vi "manual test UI.vi"(8 "error in (no error)":errorcluster caption="Fehler (Eingang, kein Fehler)", 11 "Burst Eingang":refnum<class "Burst.lvclass"> caption="DNL_LabVIEW Object in") -> (0 "error out":errorcluster caption="Fehler (Ausgang)", 1 "abbrechen":bool, 2 "Parameters":u32[](array[numeric]), 3 "Burst Ausgang":refnum<class "Burst.lvclass"> caption="DNL_LabVIEW Object out")   [LabVIEW 2013, in "Burst.lvclass"]
uses:
  Burst.lvclass
  Polaritaet.ctl
  lib/Utilities.lvlib
panel:
  in  "#OfAmps":u32=1 min=1 max=4 step=1
  in  "Amplituden (200 - 4200V) 4":u32=200 min=200 max=4200 step=10
  in  "Amplituden (200 - 4200V) 3":u32=200 min=200 max=4200 step=10
  in  "Amplituden (200 - 4200V) 2":u32=200 min=200 max=4200 step=10
  in  "Testbeschreibung":string
  in  "Testdauer (1s - 10000s)":u32=1 min=1 max=1000
  in  "Burstperiode (10ms - 2400ms)":u32=10 min=10 max=2400
  in  "Burstdauer (1 - 130ms)":u32=1 min=1 max=130
  in  "Spike-Frequenz (500Hz - 100000Hz)":u32=500 min=500 max=100000
  in  "Amplituden (200 - 4200V)":u32=200 min=200 max=4200 step=10
  in  "Einkopplung":bool
  in  "Polarität":T1
  in  "ok":bool
  in  "abbrechen 2":bool
  # "bis zu 4 verschiedne Amplituden können angegebn werden"
  # "Polarität"
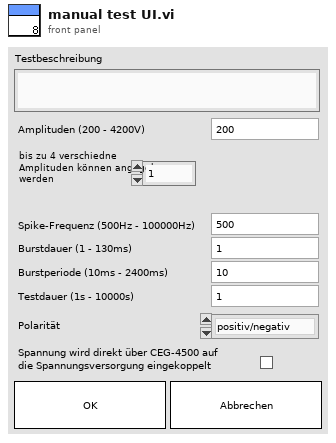
[diagram p1: front panel]
types:
  T1 = typedef "Burst.lvclass/Polaritaet.ctl" = enum16{"positiv/negativ", "negativ", "positiv"}
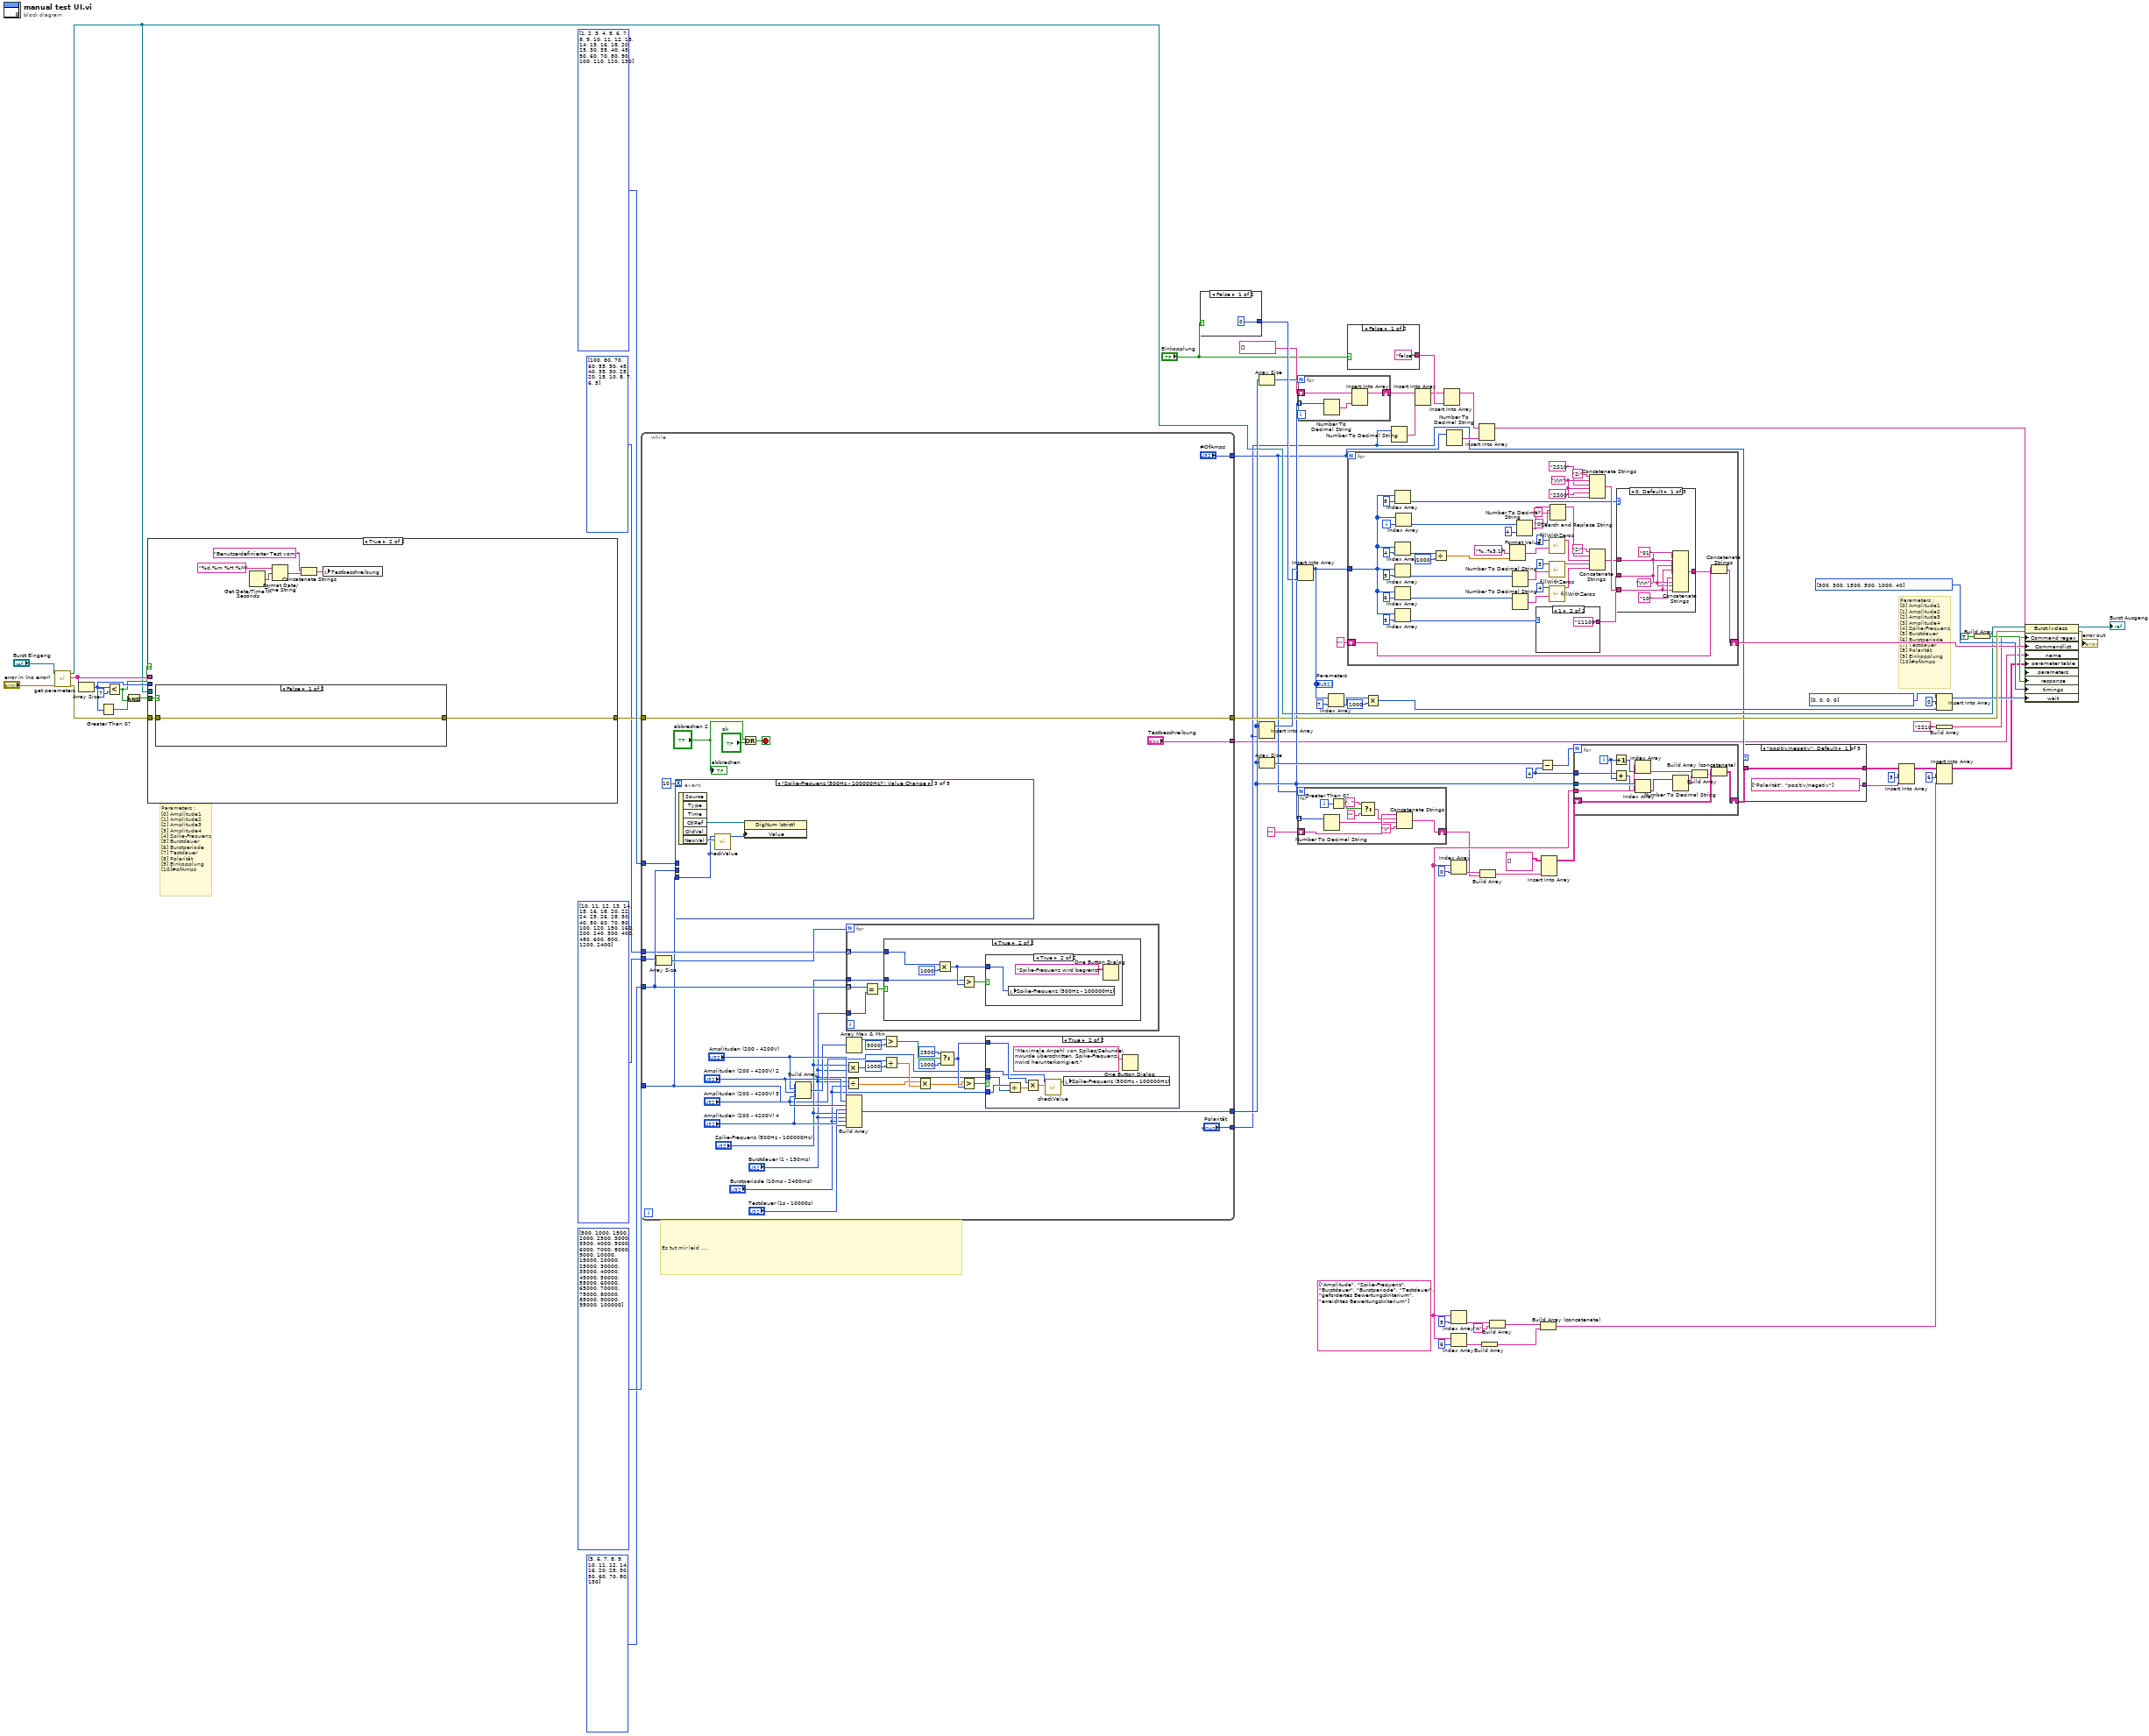
[diagram p0: block diagram]
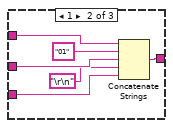
[diagram p2: hidden frame]
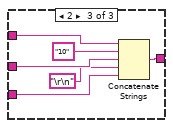
[diagram p3: hidden frame]
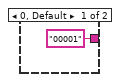
[diagram p4: hidden frame]
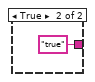
[diagram p5: hidden frame]
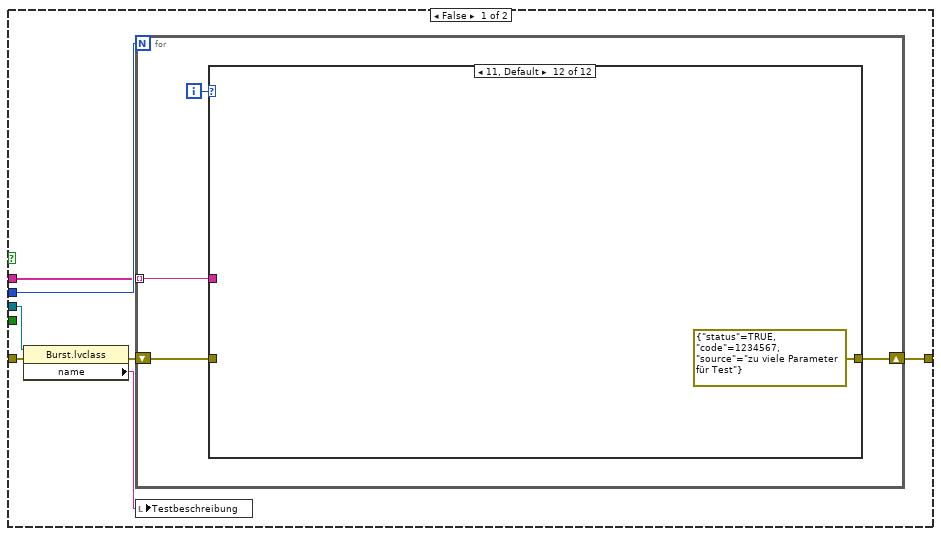
[diagram p6: hidden frame]
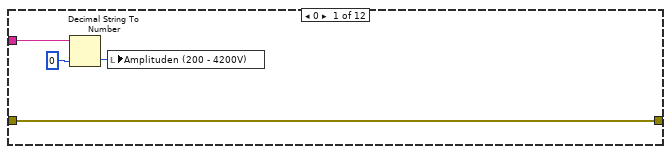
[diagram p7: hidden frame]
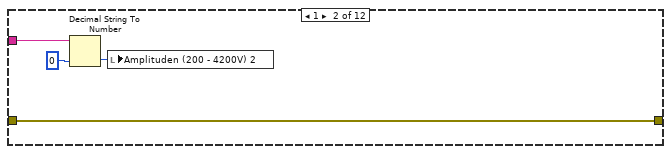
[diagram p8: hidden frame]
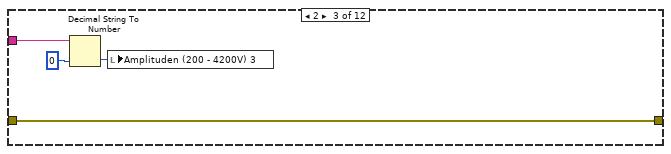
[diagram p9: hidden frame]
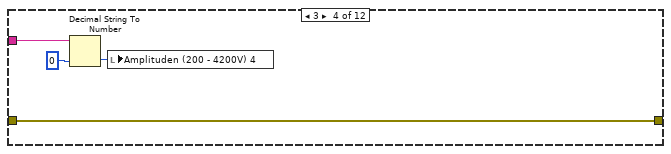
[diagram p10: hidden frame]
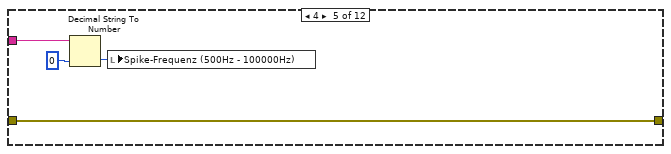
[diagram p11: hidden frame]
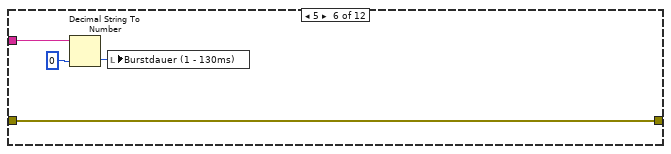
[diagram p12: hidden frame]
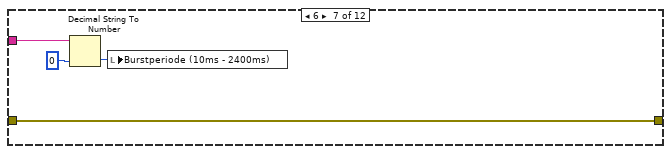
[diagram p13: hidden frame]
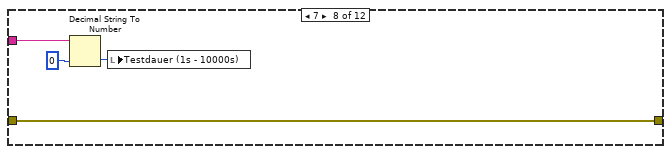
[diagram p14: hidden frame]
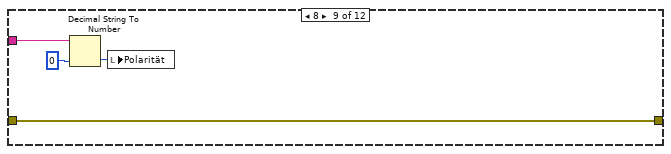
[diagram p15: hidden frame]
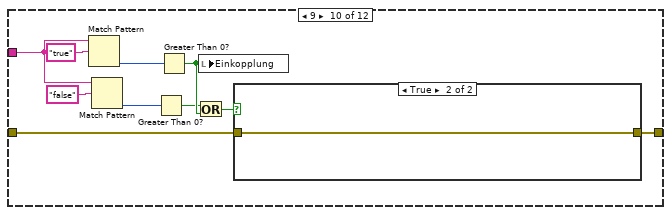
[diagram p16: hidden frame]
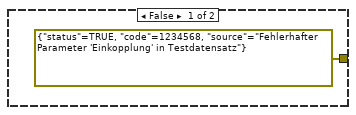
[diagram p17: hidden frame]
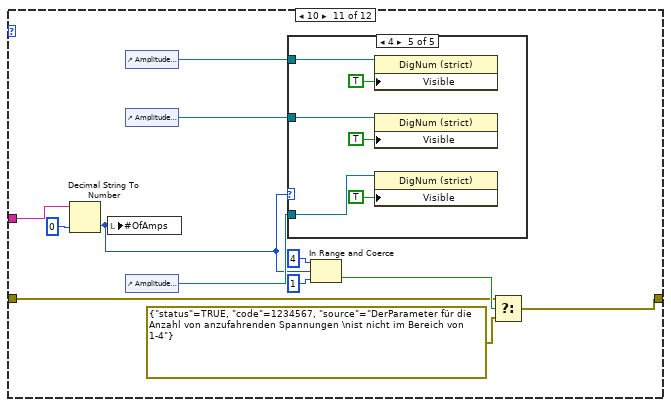
[diagram p18: hidden frame]
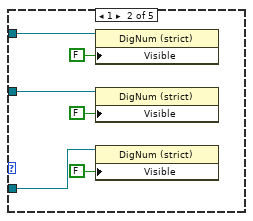
[diagram p20: hidden frame]
diagram:
  w24 = 4 ("y")
  w22 = string[] ["Amplitude", "Spike-Frequenz", "Burstdauer", "Burstperiode", "Testdauer", "gefordertes Bewertungskriterium", "erreichtes Bewertungskriterium"]
  # "Parameters :\n[0] Amplitude1\n[1] Amplitude2\n[2] Amplitude3\n[3] Amplitude4\n[4] Spike-Frequenz\n[5] Burstdauer\n[6] Burstperiode\n[7] Testdauer\n[8] Polarität\n[9] Einkopplung\n[10]#ofAmps"
  # "Parameters :\n[0] Amplitude1\n[1] Amplitude2\n[2] Amplitude3\n[3] Amplitude4\n[4] Spike-Frequenz\n[5] Burstdauer\n[6] Burstperiode\n[7] Testdauer\n[8] Polarität\n[9] Einkopplung\n[10]#ofAmps"
  # "Es tut mir leid ...."
  n1 = call-dynamic "get parameters.vi"("error in (no error)"="error in (no error)", "TestInterface (Eingang)"="Burst Eingang") -> ("error out"=w57:errorcluster, "parameters"=w58:string[], "TestInterface (Ausgang)"=w29:refnum<class "Burst.lvclass">)  [unwired: 7 in]
  n2 = Array Size(array=w58) -> (size(s)=w40:i32)
  n3 = Greater Than 0?(x=w40) -> (x > 0?=w39:bool)
  n4 = Less?(x=w40, y=7) -> (x < y?=w38:bool)
  n5 = And(x=w39, y=w38) -> (x .and. y?=w37:bool)
  n6 = case shown="True" w38 {
    tunnel: w40 -> [w83 _]
    tunnel: w58 -> [w82 _]
    tunnel: w57 -> [w79 w175]
    tunnel: [w81 w173] -> w56
    tunnel: w37 -> [_ w174]
    tunnel: w29 -> [w80 _]
    frame False {
      n7 = property class="Burst.lvclass"(reference=w80, error in=w79) -> (error out=w78:errorcluster, "name"=w77:string)  [unwired: 1 out]
      n8 = for {
        N: w83 -> [_]
        tunnel: w82 -> [w86] mode=indexing
        shift-right: [w85] -> w81
        shift-left: w78 -> [w84]
        i -> [w87]
        n9 = case shown="11, Default" w87 {
          tunnel: w86 -> [w91 w95 w99 w103 w105 w109 w113 w117 w121 w124 w146 _]
          tunnel: w84 -> [w88 w92 w96 w100 w104 w108 w112 w116 w120 w126 w142 _]
          tunnel: [w88 w92 w96 w100 w104 w108 w112 w116 w120 w128 w141 errorcluster {"status"=TRUE, "code"=1234567, "source"="zu viele Parameter für Test"} ("error constant")] -> w85
          frame 0 {
            n10 = Decimal String To Number(string=w91, default (0L)=u32 0 ("default (0 I32)")) -> (number=w90:u32)  [unwired: 1 in, 1 out]
            n11 = local write "Amplituden (200 - 4200V)"(w90) -> ()
          }
          frame 1 {
            n12 = Decimal String To Number(string=w95, default (0L)=u32 0 ("default (0 I32)")) -> (number=w94:u32)  [unwired: 1 in, 1 out]
            n13 = local write "Amplituden (200 - 4200V) 2"(w94) -> ()
          }
          frame 2 {
            n14 = Decimal String To Number(string=w99, default (0L)=u32 0 ("default (0 I32)")) -> (number=w98:u32)  [unwired: 1 in, 1 out]
            n15 = local write "Amplituden (200 - 4200V) 3"(w98) -> ()
          }
          frame 3 {
            n16 = Decimal String To Number(string=w103, default (0L)=u32 0 ("default (0 I32)")) -> (number=w102:u32)  [unwired: 1 in, 1 out]
            n17 = local write "Amplituden (200 - 4200V) 4"(w102) -> ()
          }
          frame 4 {
            n18 = Decimal String To Number(string=w105, default (0L)=u32 0 ("default (0 I32)")) -> (number=w106:u32)  [unwired: 1 in, 1 out]
            n19 = local write "Spike-Frequenz (500Hz - 100000Hz)"(w106) -> ()
          }
          frame 5 {
            n20 = Decimal String To Number(string=w109, default (0L)=u32 0 ("default (0 I32)")) -> (number=w110:u32)  [unwired: 1 in, 1 out]
            n21 = local write "Burstdauer (1 - 130ms)"(w110) -> ()
          }
          frame 6 {
            n22 = Decimal String To Number(string=w113, default (0L)=u32 0 ("default (0 I32)")) -> (number=w114:u32)  [unwired: 1 in, 1 out]
            n23 = local write "Burstperiode (10ms - 2400ms)"(w114) -> ()
          }
          frame 7 {
            n24 = Decimal String To Number(string=w117, default (0L)=u32 0 ("default (0 I32)")) -> (number=w118:u32)  [unwired: 1 in, 1 out]
            n25 = local write "Testdauer (1s - 10000s)"(w118) -> ()
          }
          frame 8 {
            n26 = Decimal String To Number(string=w121, default (0L)=u32 0 ("default (0 I32)")) -> (number=w122:u32)  [unwired: 1 in, 1 out]
            n27 = local write "Polarität"(w122) -> ()
          }
          frame 9 {
            n28 = Match Pattern(string=w124, regular expression="true") -> (offset past match=w132:i32)  [unwired: 1 in, 3 out]
            n29 = Match Pattern(string=w124, regular expression="false") -> (offset past match=w130:i32)  [unwired: 1 in, 3 out]
            n30 = Greater Than 0?(x=w130) -> (x > 0?=w127:bool)
            n31 = Greater Than 0?(x=w132) -> (x > 0?=w129:bool)
            n32 = Or(x=w127, y=w129) -> (x .or. y?=w125:bool)
            n33 = local write "Einkopplung"(w129) -> ()
            n34 = case shown="True" w125 {
              tunnel: [errorcluster {"status"=TRUE, "code"=1234568, "source"="Fehlerhafter Parameter 'Einkopplung' in Testdatensatz"} ("error constant") w135] -> w128
              tunnel: w126 -> [_ w135]
              frame False {
              }
              frame True {
              }
            }
          }
          frame 10 {
            n35 = Decimal String To Number(string=w146, default (0L)=u32 0 ("default (0 I32)")) -> (number=w136:u32)  [unwired: 1 in, 1 out]
            n36 = local write "#OfAmps"(w136) -> ()
            n37 = control-ref of="Amplituden (200 - 4200V) 4"() -> (w137:refnum<vi>)
            n38 = control-ref of="Amplituden (200 - 4200V) 2"() -> (w139:refnum<vi>)
            n39 = control-ref of="Amplituden (200 - 4200V) 3"() -> (w138:refnum<vi>)
            n40 = case shown="4" w136 {
              tunnel: w139 -> [_ w153 w159 w165 w171]
              tunnel: w138 -> [_ w149 w155 w161 w167]
              tunnel: w137 -> [_ w148 w154 w160 w166]
              frame 0, Default {
              }
              frame 1 {
                n41 = property class="DigNum (strict)"(reference=w148, "Visible"=FALSE) -> ()  [unwired: 1 in, 2 out]
                n42 = property class="DigNum (strict)"(reference=w153, "Visible"=FALSE) -> ()  [unwired: 1 in, 2 out]
                n43 = property class="DigNum (strict)"(reference=w149, "Visible"=FALSE) -> ()  [unwired: 1 in, 2 out]
              }
              frame 2 {
                n44 = property class="DigNum (strict)"(reference=w154, "Visible"=FALSE) -> ()  [unwired: 1 in, 2 out]
                n45 = property class="DigNum (strict)"(reference=w159, "Visible"=TRUE) -> ()  [unwired: 1 in, 2 out]
                n46 = property class="DigNum (strict)"(reference=w155, "Visible"=FALSE) -> ()  [unwired: 1 in, 2 out]
              }
              frame 3 {
                n47 = property class="DigNum (strict)"(reference=w160, "Visible"=FALSE) -> ()  [unwired: 1 in, 2 out]
                n48 = property class="DigNum (strict)"(reference=w165, "Visible"=TRUE) -> ()  [unwired: 1 in, 2 out]
                n49 = property class="DigNum (strict)"(reference=w161, "Visible"=TRUE) -> ()  [unwired: 1 in, 2 out]
              }
              frame 4 {
                n50 = property class="DigNum (strict)"(reference=w166, "Visible"=TRUE) -> ()  [unwired: 1 in, 2 out]
                n51 = property class="DigNum (strict)"(reference=w171, "Visible"=TRUE) -> ()  [unwired: 1 in, 2 out]
                n52 = property class="DigNum (strict)"(reference=w167, "Visible"=TRUE) -> ()  [unwired: 1 in, 2 out]
              }
            }
            n53 = In Range and Coerce(upper limit=u32 4, x=w136, lower limit=u32 1) -> (In Range?=w143:bool)  [unwired: 1 out]
            n54 = Select(t=w142, s=w143, f=errorcluster {"status"=TRUE, "code"=1234567, "source"="DerParameter für die Anzahl von anzufahrenden Spannungen \nist nicht im Bereich von 1-4"} ("error constant")) -> (s? t:f=w141:errorcluster)
          }
          frame 11, Default {
          }
        }
      }
      n55 = local write "Testbeschreibung"(w77) -> ()
    }
    frame True {
      n56 = case shown="False" w174 {
        tunnel: w175 -> [w181 _]
        tunnel: [w181 errorcluster {"status"=TRUE, "code"=123458, "source"="Der Parametersatz für den aktuellen Test ist unvollständig und\nkonnte nicht geladen werden"} ("error constant")] -> w173
        frame False {
        }
        frame True {
        }
      }
      n57 = Get Date/Time In Seconds() -> (seconds since 1Jan1904=w180:timestamp)
      n58 = Format Date/Time String(time format string (%c)="%d.%m %H:%M" ("Zeitformatierungs-String (%c)"), seconds (now)=w180) -> (date/time string=w177:string)  [unwired: 1 in]
      n59 = Concatenate Strings("Benutzerdefinierter Test vom " ("name"), w177) -> (w176:string)
      n60 = local write "Testbeschreibung"(w176) -> ()
    }
  }
  n61 = while {
    tunnel: [w214] -> w23
    tunnel: u32[] [10, 11, 12, 13, 14, 15, 16, 18, 20, 22, 24, 25, 26, 28, 30, 40, 50, 60, 70, 80, 100, 120, 150, 160, 200, 240, 300, 400, 480, 600, 800, 1200, 2400] -> [w213]
    tunnel: u32[] [500, 1000, 1500, 2000, 2500, 3000, 3500, 4000, 5000, 6000, 7000, 8000, 9000, 10000, 15000, 20000, 25000, 30000, 35000, 40000, 45000, 50000, 55000, 60000, 65000, 70000, 75000, 80000, 85000, 90000, 95000, 100000] -> [w185]
    tunnel: u32[] [1, 2, 3, 4, 5, 6, 7, 8, 9, 10, 11, 12, 13, 14, 15, 16, 18, 20, 25, 30, 35, 40, 45, 50, 60, 70, 80, 90, 100, 110, 120, 130] -> [w212]
    tunnel: w56 -> [w210]
    tunnel: [w210] -> w49
    tunnel: ["#OfAmps"] -> w5
    tunnel: ["Polarität"] -> w4
    tunnel: ["Testbeschreibung"] -> w3
    tunnel: u32[] [100, 80, 70, 60, 55, 50, 45, 40, 35, 30, 25, 20, 15, 10, 8, 7, 6, 5] -> [w204]
    tunnel: u32[] [5, 6, 7, 8, 9, 10, 11, 12, 14, 16, 20, 25, 30, 50, 60, 70, 80, 130] -> [w205]
    stop <- w218 stop-if-true
    n62 = Array Size(array=w205) -> (size(s)=w206:i32)
    n63 = event shown="[2] \"Spike-Frequenz (500Hz - 100000Hz)\": Value Change" {
      selector: _ -> [_ _ _ _ _]
      dyn-events: _ -> [_ _ _ _ _]
      timeout: 10 -> [_ _ _ _ _]
      tunnel: w213 -> [w242 _ _ _ _]
      tunnel: w185 -> [_ _ w243 _ _]
      tunnel: w212 -> [_ _ _ _ w275]
      event "Burstperiode (10ms - 2400ms)": Value Change {
        n64 = event-data() -> ("CtlRef"=w240:refnum<vi>, "NewVal"=w241:u32)  [unwired: 1 in, 4 out]
        n65 = call "checkValue.vi"("Value"=w241, "Array of valid Values"=w242) -> ("new Value"=w239:u32)  [unwired: 7 in]
        n66 = property class="DigNum (strict)"(reference=w240, "Value"=w239) -> ()  [unwired: 1 in, 2 out]
      }
      event Timeout {
        n67 = event-data() -> ()  [unwired: 1 in, 3 out]
      }
      event "Spike-Frequenz (500Hz - 100000Hz)": Value Change {
        n68 = event-data() -> ("CtlRef"=w245:refnum<vi>, "NewVal"=w244:u32)  [unwired: 1 in, 4 out]
        n69 = call "checkValue.vi"("Value"=w244, "Array of valid Values"=w243) -> ("new Value"=w246:u32)  [unwired: 7 in]
        n70 = property class="DigNum (strict)"(reference=w245, "Value"=w246) -> ()  [unwired: 1 in, 2 out]
      }
      event "#OfAmps": Value Change {
        n71 = event-data() -> ("NewVal"=w250:u32)  [unwired: 1 in, 5 out]
        n72 = control-ref of="Amplituden (200 - 4200V) 4"() -> (w247:refnum<vi>)
        n73 = control-ref of="Amplituden (200 - 4200V) 3"() -> (w248:refnum<vi>)
        n74 = control-ref of="Amplituden (200 - 4200V) 2"() -> (w249:refnum<vi>)
        n75 = case shown="4" w250 {
          tunnel: w249 -> [_ w256 w262 w268 w274]
          tunnel: w248 -> [_ w252 w258 w264 w270]
          tunnel: w247 -> [_ w251 w257 w263 w269]
          frame 0, Default {
          }
          frame 1 {
            n76 = property class="DigNum (strict)"(reference=w251, "Visible"=FALSE) -> ()  [unwired: 1 in, 2 out]
            n77 = property class="DigNum (strict)"(reference=w252, "Visible"=FALSE) -> ()  [unwired: 1 in, 2 out]
            n78 = property class="DigNum (strict)"(reference=w256, "Visible"=FALSE) -> ()  [unwired: 1 in, 2 out]
          }
          frame 2 {
            n79 = property class="DigNum (strict)"(reference=w257, "Visible"=FALSE) -> ()  [unwired: 1 in, 2 out]
            n80 = property class="DigNum (strict)"(reference=w258, "Visible"=FALSE) -> ()  [unwired: 1 in, 2 out]
            n81 = property class="DigNum (strict)"(reference=w262, "Visible"=TRUE) -> ()  [unwired: 1 in, 2 out]
          }
          frame 3 {
            n82 = property class="DigNum (strict)"(reference=w263, "Visible"=FALSE) -> ()  [unwired: 1 in, 2 out]
            n83 = property class="DigNum (strict)"(reference=w264, "Visible"=TRUE) -> ()  [unwired: 1 in, 2 out]
            n84 = property class="DigNum (strict)"(reference=w268, "Visible"=TRUE) -> ()  [unwired: 1 in, 2 out]
          }
          frame 4 {
            n85 = property class="DigNum (strict)"(reference=w269, "Visible"=TRUE) -> ()  [unwired: 1 in, 2 out]
            n86 = property class="DigNum (strict)"(reference=w270, "Visible"=TRUE) -> ()  [unwired: 1 in, 2 out]
            n87 = property class="DigNum (strict)"(reference=w274, "Visible"=TRUE) -> ()  [unwired: 1 in, 2 out]
          }
        }
      }
      event "Burstdauer (1 - 130ms)": Value Change {
        n88 = event-data() -> ("CtlRef"=w277:refnum<vi>, "NewVal"=w276:u32)  [unwired: 1 in, 4 out]
        n89 = call "checkValue.vi"("Value"=w276, "Array of valid Values"=w275) -> ("new Value"=w278:u32)  [unwired: 7 in]
        n90 = property class="DigNum (strict)"(reference=w277, "Value"=w278) -> ()  [unwired: 1 in, 2 out]
      }
    }
    n91 = Or(x="abbrechen 2", y="ok") -> (x .or. y?=w218:bool)
    n92 = Build Array("Amplituden (200 - 4200V) 4", "Amplituden (200 - 4200V)", "Amplituden (200 - 4200V) 2", "Amplituden (200 - 4200V) 3") -> (w199:u32[])
    n93 = Multiply(x="Spike-Frequenz (500Hz - 100000Hz)", y="Burstdauer (1 - 130ms)") -> (x*y=w190:u32)
    n94 = Divide(x="Burstdauer (1 - 130ms)", y="Burstperiode (10ms - 2400ms)") -> (x/y=w193:dbl)
    n95 = for {
      N: w206 -> [_]
      tunnel: w205 -> [w231] mode=indexing
      tunnel: "Burstdauer (1 - 130ms)" -> [w230]
      tunnel: w204 -> [w228] mode=indexing
      tunnel: "Spike-Frequenz (500Hz - 100000Hz)" -> [w227]
      n96 = Equal?(x=w231, y=w230) -> (x = y?=w229:bool)
      n97 = case shown="True" w229 {
        tunnel: w228 -> [_ w236]
        tunnel: w227 -> [_ w232]
        frame False {
        }
        frame True {
          n98 = Multiply(x=w236, y=u32 1000) -> (x*y=w233:u32)
          n99 = Greater?(x=w232, y=w233) -> (0:w234:bool)
          n100 = case shown="True" w234 {
            tunnel: w233 -> [_ w238]
            frame False {
            }
            frame True {
              n101 = local write "Spike-Frequenz (500Hz - 100000Hz)"(w238) -> ()
              n102 = One Button Dialog(message="Spike-Frequenz wird begrenzt") -> ()  [unwired: 1 in, 1 out]
            }
          }
        }
      }
    }
    n103 = Array Max & Min(array=w199) -> (max value=w198:u32)  [unwired: 3 out]
    n104 = Build Array("Amplituden (200 - 4200V)", "Amplituden (200 - 4200V) 2", "Amplituden (200 - 4200V) 3", "Amplituden (200 - 4200V) 4", "Spike-Frequenz (500Hz - 100000Hz)", "Burstdauer (1 - 130ms)", "Burstperiode (10ms - 2400ms)", "Testdauer (1s - 10000s)") -> (w214:u32[])
    n105 = Greater?(x=w198, y=u32 3000) -> (0:w196:bool)
    n106 = Divide(x=w190, y=u32 1000) -> (x/y=w191:dbl)
    n107 = Multiply(x=w193, y=w191) -> (x*y=w188:dbl)
    n108 = Select(t=u32 2500, s=w196, f=u32 1000) -> (s? t:f=w186:u32)
    n109 = Greater?(x=w188, y=w186) -> (0:w187:bool)
    n110 = case shown="True" w187 {
      tunnel: w186 -> [_ w225]
      tunnel: "Burstdauer (1 - 130ms)" -> [_ w219]
      tunnel: "Burstperiode (10ms - 2400ms)" -> [_ w220]
      tunnel: w185 -> [_ w223]
      frame False {
      }
      frame True {
        n111 = Divide(x=w220, y=w219) -> (x/y=w224:dbl)
        n112 = Multiply(x=w225, y=w224) -> (x*y=w221:dbl)
        n113 = call "checkValue.vi"("Value"=w221, "Array of valid Values"=w223) -> ("new Value"=w222:u32)  [unwired: 7 in]
        n114 = local write "Spike-Frequenz (500Hz - 100000Hz)"(w222) -> ()
        n115 = One Button Dialog(message="Maximale Anzahl von Spikes/Sekunde\nwurde überschritten. Spike-Frequenz\nwird herunterkorrigiert.") -> ()  [unwired: 1 in, 1 out]
      }
    }
    "abbrechen" <- "abbrechen 2"
  }
  n116 = case shown="False" "Einkopplung" {
    tunnel: [u32 0 u32 1] -> w75
    frame False {
    }
    frame True {
    }
  }
  n117 = Array Size(array=w23) -> (size(s)=w33:i32)
  n118 = Insert Into Array(array=w23, new element=w4) -> (w76:u32[])  [unwired: 1 in]
  n119 = Array Size(array=w23) -> (size(s)=w26:i32)
  n120 = for {
    N: w33 -> [_]
    tunnel: w23 -> [w284] mode=indexing
    shift-right: [w281] -> w10
    shift-left: string[] [] -> [w282]
    n121 = Number To Decimal String(number=w284) -> (decimal integer string=w283:string)  [unwired: 1 in]
    n122 = Insert Into Array(array=w282, new element=w283) -> (w281:string[])  [unwired: 1 in]
  }
  n123 = Insert Into Array(array=w76, new element=w75) -> (w27:u32[])  [unwired: 1 in]
  "Parameters" <- w27
  n124 = for {
    N: w5 -> [_]
    tunnel: w23 -> [w294] mode=indexing
    shift-right: [w285] -> w19
    shift-left: "" -> [w289]
    i -> [w293]
    n125 = Number To Decimal String(number=w294) -> (decimal integer string=w287:string)  [unwired: 1 in]
    n126 = Greater Than 0?(x=w293) -> (x > 0?=w292:bool)
    n127 = Select(t=", ", s=w292, f="") -> (s? t:f=w288:string)
    n128 = Concatenate Strings(w289, w288, w287, "V" ("string")) -> (w285:string)
  }
  n129 = Index Array(array=w27, index=7) -> (element=w53:u32)
  n130 = case shown="False" "Einkopplung" {
    tunnel: ["false" "true"] -> w30
    frame False {
    }
    frame True {
    }
  }
  n131 = for {
    N: w5 -> [_]
    tunnel: w27 -> [w301]
    shift-right: [w300] -> w46
    shift-left: "" -> [w299]
    i -> [w297]
    w336 = "\r\n"
    n132 = Index Array(array=w301, index=8) -> (element=w330:u32)
    n133 = Index Array(array=w301, index=4) -> (element=w310:u32)
    n134 = Index Array(array=w301, index=5) -> (element=w318:u32)
    n135 = Index Array(array=w301, index=6) -> (element=w324:u32)
    n136 = Index Array(array=w301, index=9) -> (element=w329:u32)
    n137 = Index Array(array=w301, index=w297) -> (element=w303:u32)
    n138 = Divide(x=w310, y=u32 1000) -> (x/y=w312:dbl)
    n139 = Format Value(format string="%.;%3.1f", value (0)=w312) -> (output string=w315:string)  [unwired: 1 in]
    n140 = Number To Decimal String(number=w318) -> (decimal integer string=w319:string)  [unwired: 1 in]
    n141 = Number To Decimal String(number=w324) -> (decimal integer string=w323:string)  [unwired: 1 in]
    n142 = Number To Decimal String(number=w303, width (-)=i16 4) -> (decimal integer string=w305:string)
    n143 = case shown="1" w329 {
      tunnel: ["00001" "11100"] -> w332
      frame 0, Default {
      }
      frame 1 {
      }
    }
    n144 = call "fillWithZeros.vi"("string in"=w315, "width"=5 ("x")) -> ("string out"=w316:string)  [unwired: 9 in]
    n145 = call "fillWithZeros.vi"("string in"=w319, "width"=3) -> ("string out"=w321:string)  [unwired: 9 in]
    n146 = call "fillWithZeros.vi"("string in"=w323, "width"=4) -> ("string out"=w326:string)  [unwired: 9 in]
    n147 = Search and Replace String(input string=w305, search string=" ", replace string="0" ("replace string (\"\")")) -> (result string=w308:string)  [unwired: 5 in, 3 out]
    n148 = Concatenate Strings("2i" ("String"), w336, "2S10", w336, "2S00", w336) -> (w337:string)
    n149 = Concatenate Strings("2I", w308, w316, w321, w326) -> (w331:string)
    n150 = case shown="0, Default" w330 {
      tunnel: w331 -> [w342 w350 w356]
      tunnel: w332 -> [w340 w348 w355]
      tunnel: [w343 w347 w353] -> w298
      tunnel: w337 -> [w339 w345 w351]
      frame 0, Default {
        w338 = "\r\n"
        n151 = Concatenate Strings(w342, "01" ("string"), w340, w338, w339, w342, "10" ("string"), w340, w338, w339) -> (w343:string)
      }
      frame 1 {
        n152 = Concatenate Strings(w350, "01" ("string"), w348, "\r\n", w345) -> (w347:string)
      }
      frame 2 {
        n153 = Concatenate Strings(w356, "10" ("string"), w355, "\r\n", w351) -> (w353:string)
      }
    }
    n154 = Concatenate Strings(w299, w298) -> (w300:string)
  }
  n155 = Multiply(x=w53, y=u32 1000) -> (x*y=w55:u32)
  n156 = Number To Decimal String(number=w4) -> (decimal integer string=w9:string)  [unwired: 1 in]
  n157 = Insert Into Array(array=w10, new element=w9) -> (w11:string[])  [unwired: 1 in]
  n158 = Insert Into Array(array=w11, new element=w30) -> (w7:string[])  [unwired: 1 in]
  n159 = Number To Decimal String(number=w5) -> (decimal integer string=w8:string)  [unwired: 1 in]
  n160 = Index Array(array=w22, index=0) -> (element=w20:string)
  n161 = Index Array(array=w22, index=5 ("Index")) -> (element=w65:string)
  n162 = Index Array(array=w22, index=6 ("Index")) -> (element=w66:string)
  n163 = Insert Into Array(array=w7, new element=w8) -> (w6:string[])  [unwired: 1 in]
  n164 = Build Array(w20, w19) -> (w14:string[])
  n165 = Build Array(w66) -> (w16:string[])
  n166 = Build Array(w65, "A" ("Element")) -> (w17:string[])
  n167 = Subtract(x=w26, y=w24) -> (x-y=w25:i32)
  n168 = Build Array (concatenate)(w17, w16) -> (w15:string[])
  n169 = Insert Into Array(array=string[][] [], new element=w14) -> (w12:string[][])  [unwired: 2 in]
  n170 = for {
    N: w25 -> [_]
    shift-right: [w367] -> w71
    shift-left: w12 -> [w369]
    tunnel: w23 -> [w366]
    tunnel: w24 -> [w364]
    tunnel: w22 -> [w363]
    i -> [w359]
    n171 = Increment(x=w359) -> (x+1=w360:i32)
    n172 = Add(x=w364, y=w359) -> (x+y=w362:i32)
    n173 = Index Array(array=w363, index=w360) -> (element=w361:string)
    n174 = Index Array(array=w366, index=w362) -> (element=w365:u32)
    n175 = Number To Decimal String(number=w365) -> (decimal integer string=w370:string)  [unwired: 1 in]
    n176 = Build Array(w361, w370) -> (w368:string[])
    n177 = Build Array (concatenate)(w369, w368) -> (w367:string[][])
  }
  n178 = case shown="\"positiv/negativ\", Default" w4 {
    tunnel: [string[] ["Polarität", "positiv/negativ"] string[] ["Polarität", "positiv"] string[] ["Polarität", "negativ"]] -> w72
    tunnel: w71 -> [w372 w374 w376]
    tunnel: [w372 w374 w376] -> w74
    frame "positiv/negativ", Default {
    }
    frame "positiv" {
    }
    frame "negativ" {
    }
  }
  n179 = Insert Into Array(array=w74, index (row)=5, new element=w72) -> (w70:string[][])  [unwired: 1 in]
  n180 = Insert Into Array(array=i32[] [0, 0, 0, 0] ("Timings"), index=0, new element=w55) -> (w48:i32[])
  n181 = Insert Into Array(array=w70, index (row)=6 ("Index (Zeile)"), new element=w15) -> (w36:string[][])  [unwired: 1 in]
  n182 = Build Array("2S10") -> (w42:string[])
  n183 = Build Array(TRUE) -> (w43:bool[])
  n184 = property class="Burst.lvclass"(reference=w29, error in=w49, "Command regex"=w42, "Commandlist"=w46, "name"=w3, "parameter table"=w36, "parameters"=w6, "response"=w43, "timings"=u32[] [300, 300, 1500, 500, 1000, 40] ("Timings"), "wait"=w48) -> (reference out=→"Burst Ausgang":refnum<class "Burst.lvclass">, error out=→"error out":errorcluster)
